vi "multimode-acquisition.vi"() -> ()   [LabVIEW 2014]
panel:
  in  "Go":bool
  in  "Quit":bool
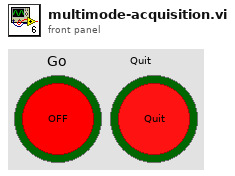
[diagram p1: front panel]
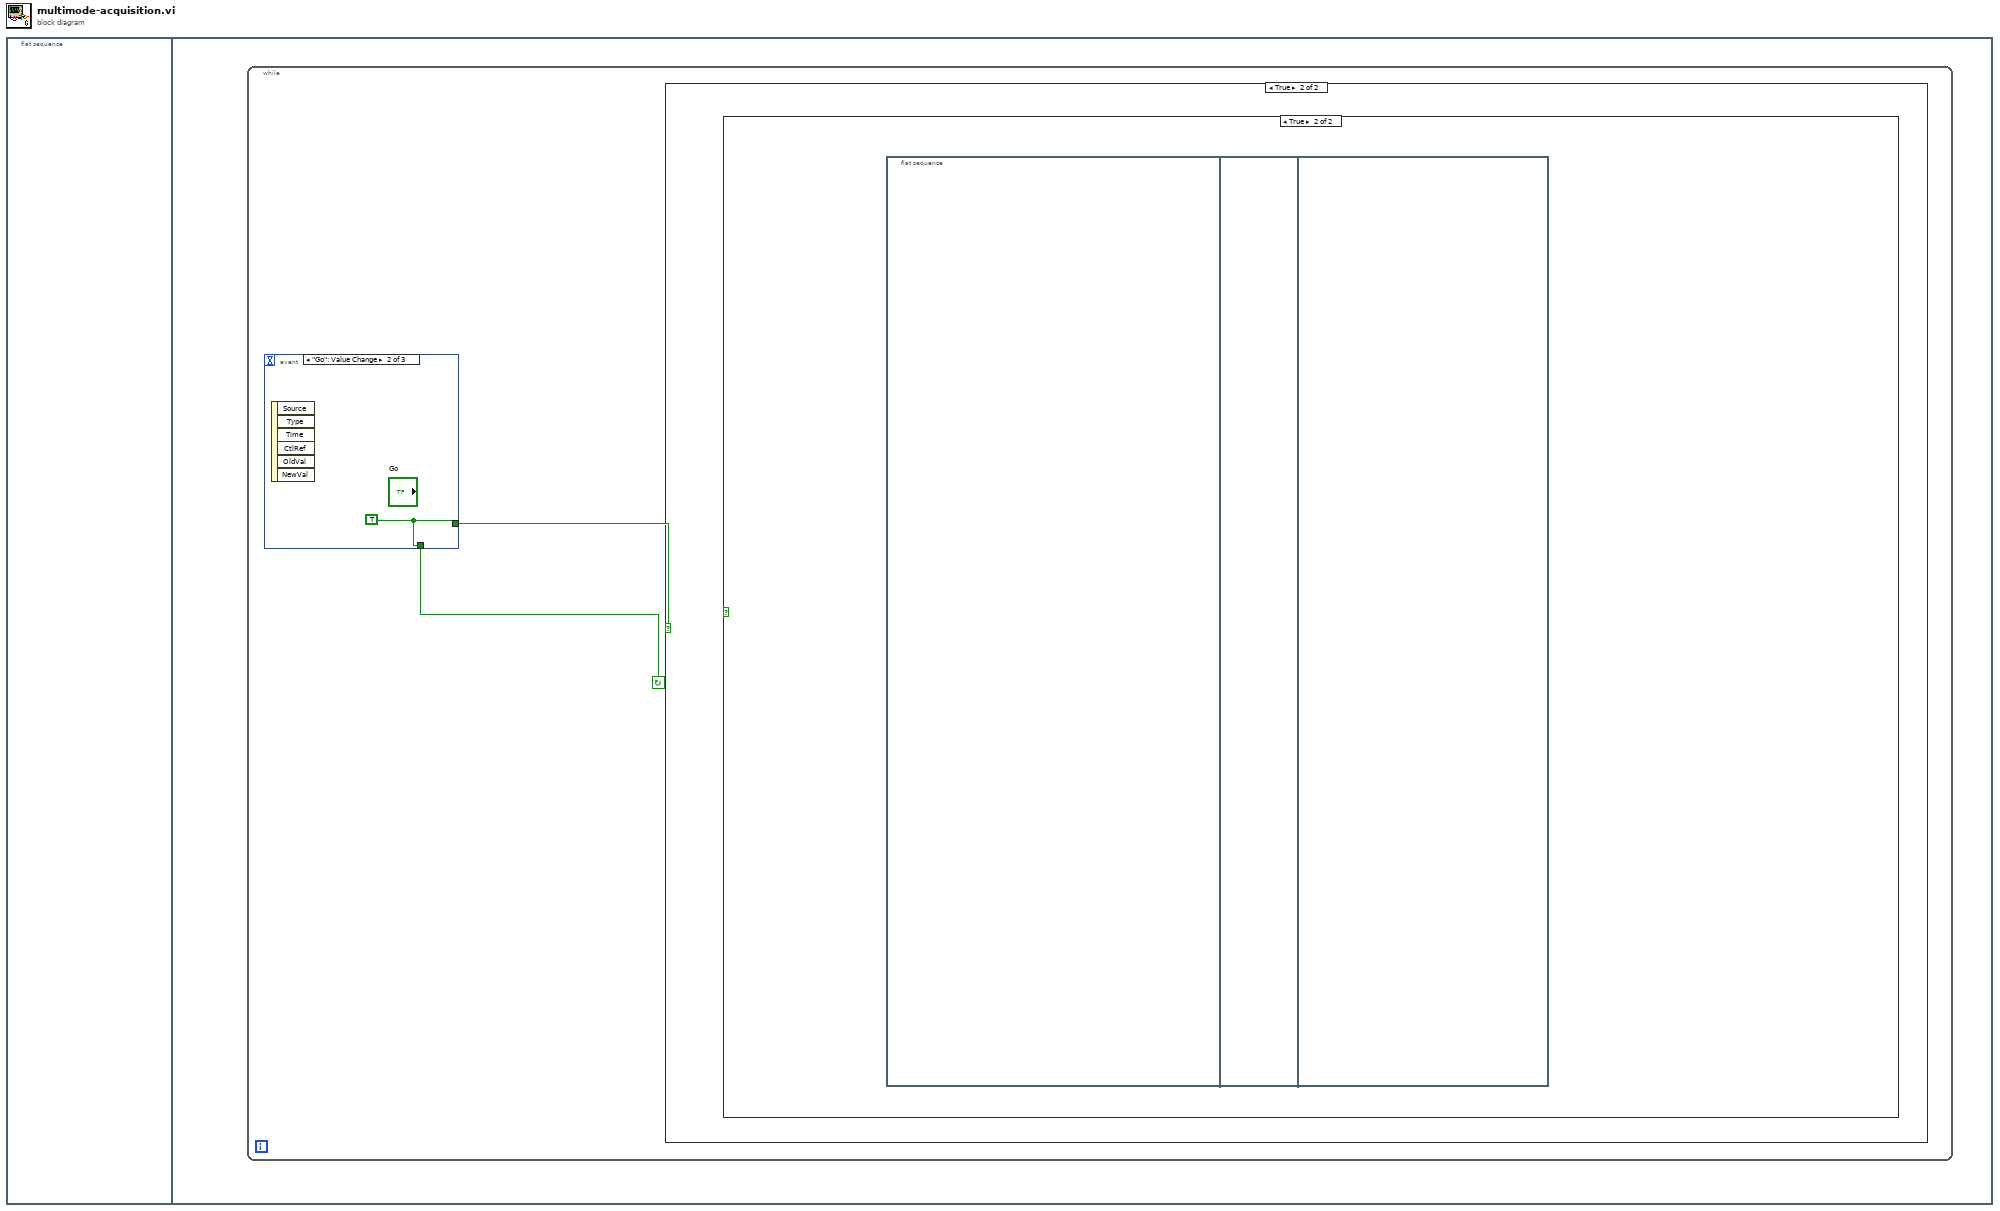
[diagram p0: block diagram]
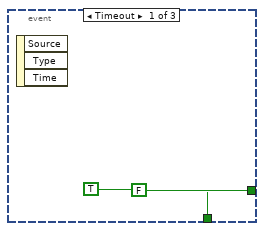
[diagram p4: hidden frame]
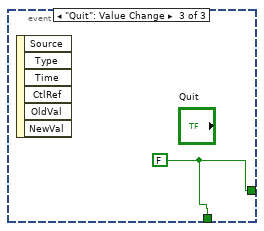
[diagram p5: hidden frame]
diagram:
  n1 = flat-sequence {
    frame #0 {
    }
    frame #1 {
      n2 = while {
        stop <- w1 continue-if-true
        n3 = event shown="[1] \"Go\": Value Change" {
          selector: _ -> [_ _ _]
          dyn-events: _ -> [_ _ _]
          timeout: _ -> [_ _ _]
          tunnel: [FALSE w5 w6] -> w2
          tunnel: [TRUE w5 w6] -> w1
          event Timeout {
            n4 = event-data() -> ()  [unwired: 1 in, 3 out]
          }
          event "Go": Value Change {
            w5 = TRUE
            n5 = event-data() -> ()  [unwired: 1 in, 6 out]
          }
          event "Quit": Value Change {
            w6 = FALSE
            n6 = event-data() -> ()  [unwired: 1 in, 6 out]
          }
        }
        n7 = case shown="True" w2 {
          frame False {
          }
          frame True {
            n8 = case shown="True" {
              selector: _ -> [_ _]
              frame False {
              }
              frame True {
                n9 = flat-sequence {
                  frame #0 {
                  }
                  frame #1 {
                  }
                  frame #2 {
                  }
                }
              }
            }
          }
        }
      }
    }
  }
